vi "Draw_Cage_Outline_(donut).vi"(0 "Picture refnum in":T1, 1 "Bounding rectangle for cage outline, pix":T2, 2 "Background color":u32(colorbox), 3 "Error In":errorcluster, 4 "Inner donut scale factor":dbl=0.56 format="%#_13g") -> (5 "Picture refnum out":T1, 7 "Error Out":errorcluster)   [LabVIEW 2018, in "Cage Diagram.lvlib"]
uses:
  Cage Diagram.lvlib
  <vilib>/vision/Image Controls.llb/IMAQ Image.ctl
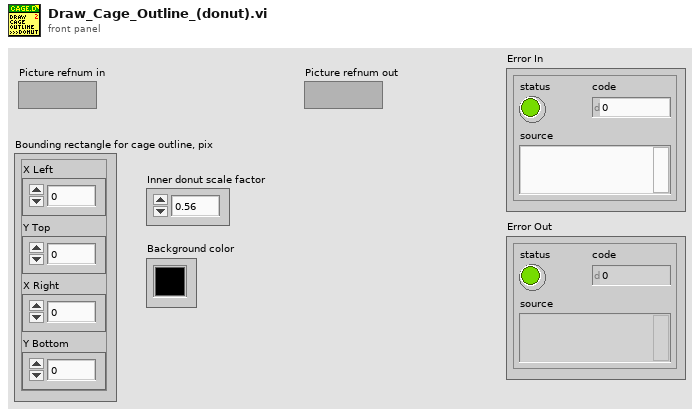
[diagram p1: front panel]
types:
  T1 = typedef "IMAQ Image.ctl" = refnum<image>
  T2 = cluster{"X Left":i32, "Y Top":i32, "X Right":i32, "Y Bottom":i32}
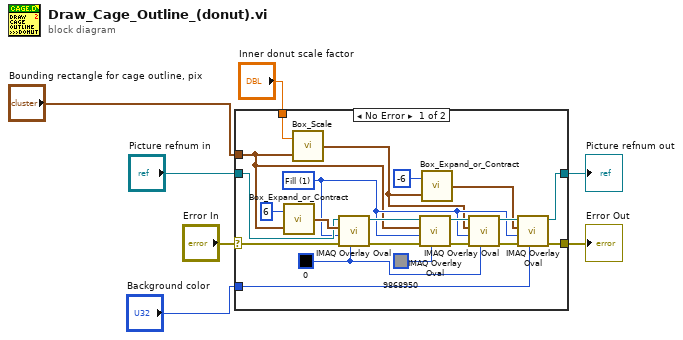
[diagram p0: block diagram]
diagram:
  n1 = case shown="No Error" "Error In" {
    selector: "Error In" -> [w26 w29]
    tunnel: [w20 w30] -> w6
    tunnel: "Picture refnum in" -> [w27 w30]
    tunnel: "Bounding rectangle for cage outline, pix" -> [w10 _]
    tunnel: [w25 w29] -> w3
    tunnel: "Background color" -> [w9 _]
    tunnel: "Inner donut scale factor" -> [w8 _]
    frame No Error {
      w19 = u32 0 ("Color")
      w15 = u32 1 items=["Frame", "Fill"] ("Drawing Mode (Frame)")
      n2 = call "Box_Expand_or_Contract.vi"("Rectangle in"=w10, "Expand/Contract"=6) -> ("Rectangle out"=w28:T2)
      n3 = call "Box_Scale.vi"("Rectangle in"=w10, "Scale factor"=w8) -> ("Rectangle out"=w11:T2)
      n4 = call "IMAQ Overlay Oval"("Color"=w19, "error in (no error)"=w26, "Drawing Mode (Frame)"=w15, "Bounding Rectangle"=w28, "Image"=w27) -> ("error out"=w17:errorcluster, "Image Out"=w18:T1)  [unwired: 5 in]
      n5 = call "IMAQ Overlay Oval"("Color"=u32 9868950, "error in (no error)"=w17, "Drawing Mode (Frame)"=w15, "Bounding Rectangle"=w10, "Image"=w18) -> ("error out"=w24:errorcluster, "Image Out"=w22:T1)  [unwired: 5 in]
      n6 = call "Box_Expand_or_Contract.vi"("Rectangle in"=w11, "Expand/Contract"=-6) -> ("Rectangle out"=w12:T2)
      n7 = call "IMAQ Overlay Oval"("Color"=w19, "error in (no error)"=w24, "Drawing Mode (Frame)"=w15, "Bounding Rectangle"=w11, "Image"=w22) -> ("error out"=w23:errorcluster, "Image Out"=w21:T1)  [unwired: 5 in]
      n8 = call "IMAQ Overlay Oval"("Color"=w9, "error in (no error)"=w23, "Drawing Mode (Frame)"=w15, "Bounding Rectangle"=w12, "Image"=w21) -> ("error out"=w25:errorcluster, "Image Out"=w20:T1)  [unwired: 5 in]
    }
    frame Error {
    }
  }
  "Error Out" <- w3
  "Picture refnum out" <- w6
